vi "RunningSum.vi"(7 "LabVIEW Web Service Request":refnum<class "Web Request.lvclass">, 10 "newNum":dbl format="%#_13g", 11 "mode":string) -> (2 "value":string, 3 "sum":dbl format="%#_13g")   [LabVIEW 2017]
uses:
  <vilib>/wsapi/Web Request.lvclass
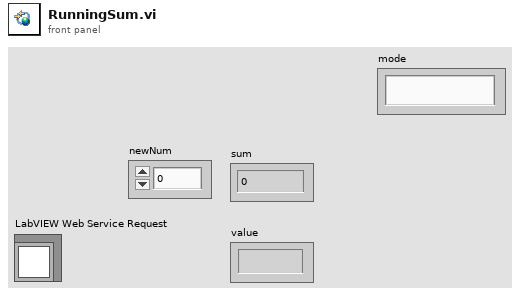
[diagram p1: front panel]
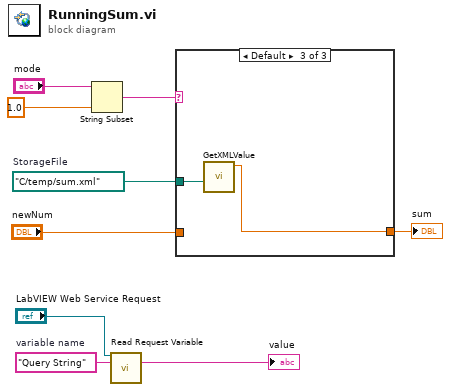
[diagram p0: block diagram]
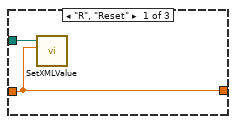
[diagram p2: hidden frame]
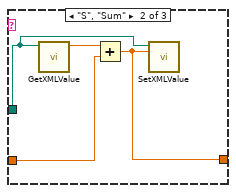
[diagram p3: hidden frame]
diagram:
  w6 = path "C:/temp/sum.xml"  # StorageFile
  w7 = "Query String"  # variable name
  n1 = String Subset(string="mode", length (rest)=1.0) -> (substring=w1:string)  [unwired: 1 in]
  n2 = call <vilib>:"Read Request Variable.vi"("LabVIEW Web Service Request"="LabVIEW Web Service Request", "variable name"=w7) -> ("value"=→"value":string)  [unwired: 11 in, 2 out]
  n3 = case shown="Default" w1 {
    tunnel: w6 -> [w11 w13 w17]
    tunnel: [w10 w12 w16] -> w5
    tunnel: "newNum" -> [w10 w14 _]
    frame "R", "Reset" {
      n4 = call "SetXMLValue.vi"("Value"=w10, "Path"=w11) -> ()  [unwired: 10 in]
    }
    frame "S", "Sum" {
      n5 = call "GetXMLValue.vi"("Path"=w13) -> ("Value"=w15:dbl)  [unwired: 10 in]
      n6 = Add(x=w15, y=w14) -> (x+y=w12:dbl)
      n7 = call "SetXMLValue.vi"("Value"=w12, "Path"=w13) -> ()  [unwired: 10 in]
    }
    frame Default {
      n8 = call "GetXMLValue.vi"("Path"=w17) -> ("Value"=w16:dbl)  [unwired: 10 in]
    }
  }
  "sum" <- w5
